vi "Create Test Sequence File.vi"() -> ()   [LabVIEW 2015]
uses:
  Prototype/classes/Sequence/Config/Sequence Config.lvclass
  Prototype/testing/Sequencer Module tests.lvlib
panel:
  out "error out":errorcluster
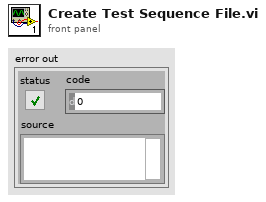
[diagram p1: front panel]
types:
  T1 = enum16{"open", "replace", "create", "open or create", "replace or create", "replace or create with confirmation"}
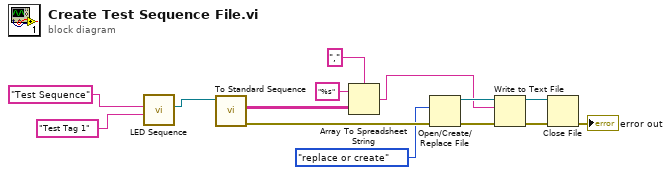
[diagram p0: block diagram]
diagram:
  n1 = call "LED Sequence.vi"("Tag Name"="Test Tag 1", "Name"="Test Sequence") -> ("Sequence out"=w11:refnum<class "Sequence Config.lvclass">)  [unwired: 9 in]
  n2 = call-dynamic "To Standard Sequence.vi"("Sequence Config in"=w11) -> ("error out"=w12:errorcluster, "Standard Sequence"=w14:string[][])  [unwired: 8 in, 1 out]
  n3 = Array To Spreadsheet String(delimiter (Tab)=",", array=w14, 3:"%s" ("format string")) -> (spreadsheet string=w6:string)
  n4 = Open/Create/Replace File(error in=w12, operation (0:open)=T1."replace or create") -> (refnum out=w7:refnum<file>, error out=w8:errorcluster)  [unwired: 4 in, 1 out]
  n5 = Write to Text File(file (use dialog)=w7, text=w6, error in=w8) -> (refnum out=w3:refnum<file>, error out=w4:errorcluster)  [unwired: 1 in, 1 out]
  n6 = Close File(refnum=w3, error in=w4) -> (error out=→"error out":errorcluster)  [unwired: 1 out]
